vi "OAT Verify Resampled Signal (OMP, Single Channel).vi"(0 "resampled signal":cluster{"r0":dbl, "dr":dbl, "Y":dbl[]} {"r0" format="%.2p"; "dr" format="%.2p"; "Y" format="%.2f"}, 1 "reset in (T)":bool=TRUE, 5 "X axis selection":u16(ring)=2 items=["Time", "Revolution", "RPM"], 7 "orders to compute (1.0)":dbl[](array[numeric])=[1.0] format="%.2f", 9 "bandwidth [order]":dbl=1.0 format="%.2f", 11 "error in (no error)":errorcluster) -> (3 "reset out (T)":bool=TRUE, 4 "resampled signal dup":cluster{"r0":dbl, "dr":dbl, "Y":dbl[]} {"r0" format="%.2p"; "dr" format="%.2p"; "Y" format="%.2f"}, 6 "X axis selection out":u16(ring)=2 items=["Time", "Revolution", "RPM"], 8 "orders to compute (1.0) out":dbl[](array[numeric])=[1.0] format="%.2f", 10 "bandwidth [order] out":dbl=1.0 format="%.2f", 15 "error out":errorcluster)   [LabVIEW 2017, in "SoundVib_Resampling.lvlib"]
uses:
  <vilib>/addons/Sound and Vibration/Order Analysis/Resample Order Tracking/SoundVib_Resampling.lvlib
  <vilib>/addons/Sound and Vibration/Order Analysis/Resample Order Tracking/SubVIs/OAT Verify Resampled Signal (Single Channel).vi
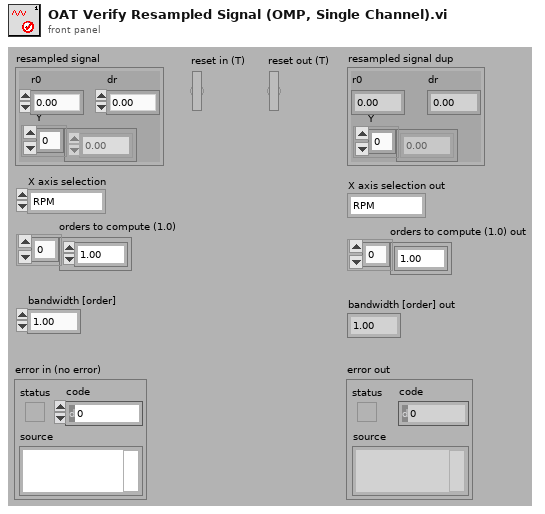
[diagram p1: front panel]
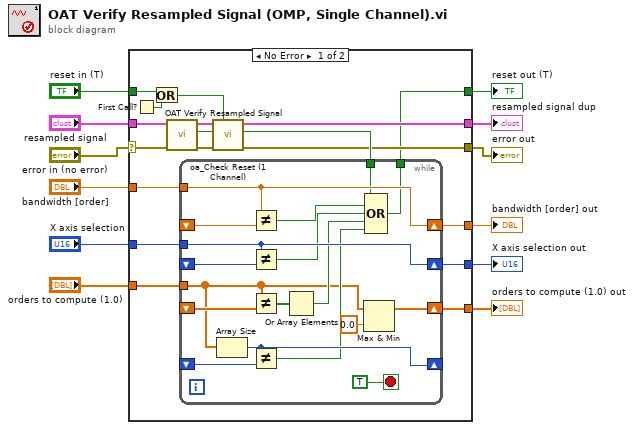
[diagram p0: block diagram]
diagram:
  n1 = case shown="No Error" "error in (no error)" {
    selector: "error in (no error)" -> [w22 w54]
    tunnel: [w19 w54] -> w11
    tunnel: "resampled signal" -> [w24 w52]
    tunnel: "bandwidth [order]" -> [w30 w51]
    tunnel: "X axis selection" -> [w29 w50]
    tunnel: "orders to compute (1.0)" -> [w28 w49]
    tunnel: "reset in (T)" -> [w27 w53]
    tunnel: [w18 w52] -> w5
    tunnel: [w17 w49] -> w4
    tunnel: [w16 w50] -> w3
    tunnel: [w15 w51] -> w2
    tunnel: [w13 w53] -> w1
    frame No Error {
      n2 = First Call?() -> (First Call?: T/F=w26:bool)
      n3 = Or(x=w27, y=w26) -> (x .or. y?=w25:bool)
      n4 = call-poly <vilib>:"OAT Verify Resampled Signal.vi"("error in (no error)"=w22, "resampled signal"=w24) -> ("error out"=w21:errorcluster, "empty signal?"=w14:bool, "resampled signal dup"=w23:cluster{"r0":dbl, "dr":dbl, "Y":dbl[]})  [unwired: 7 in]
      n5 = call <vilib>:"oa_Check Reset (1 Channel).vi"("reset?"=w25, "error in (no error)"=w21, "empty signal?"=w14, "resampled signal"=w23) -> ("error out"=w19:errorcluster, "reset out?"=w20:bool, "resampled signal dup"=w18:cluster{"r0":dbl, "dr":dbl, "Y":dbl[]})  [unwired: 5 in]
      n6 = while {
        tunnel: w30 -> [w46]
        shift-right: [w46] -> w15
        shift-left: _ -> [w47]
        shift-right: [w44] -> w16
        shift-left: _ -> [w45]
        tunnel: w29 -> [w44]
        tunnel: w28 -> [w35]
        shift-right: [w33] -> w17
        shift-left: _ -> [w43]
        shift-right: [w40] -> _
        shift-left: _ -> [w41]
        tunnel: w20 -> [w32]
        tunnel: [w31] -> w13
        stop <- TRUE stop-if-true
        n7 = Array Size(array=w35) -> (size(s)=w40:i32)
        n8 = Not Equal?(x=w46, y=w47) -> (x != y?=w39:bool)
        n9 = Not Equal?(x=w44, y=w45) -> (x != y?=w38:bool)
        n10 = Not Equal?(x=w35, y=w43) -> (x != y?=w42:bool[])
        n11 = Not Equal?(x=w40, y=w41) -> (x != y?=w36:bool)
        n12 = Or Array Elements(Boolean array=w42) -> (logical OR=w37:bool)
        n13 = Max & Min(x=w35, y=0.0) -> (max(x,y)=w33:dbl[])  [unwired: 1 out]
        n14 = Compound Arithmetic op=OR(w32, w39, w38, w37, w36) -> (w31:bool)
      }
    }
    frame Error {
    }
  }
  "error out" <- w11
  "resampled signal dup" <- w5
  "reset out (T)" <- w1
  "bandwidth [order] out" <- w2
  "orders to compute (1.0) out" <- w4
  "X axis selection out" <- w3
